vi "Boiler Controller.vi"() -> ()   [LabVIEW 2015]
uses:
  support/Message Queue/All Message Queues.ctl
  support/Message Queue/Message Cluster.ctl
  support/Message Queue/Message Queue.lvlib
panel:
  out "Error Out":errorcluster
  in  "Error In":errorcluster
  in  "Message Queues":T1
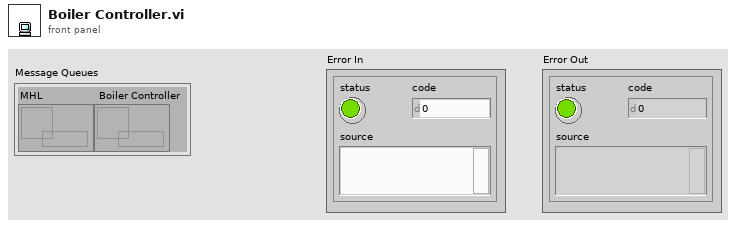
[diagram p1: front panel]
types:
  T1 = typedef "Message Queue.lvlib/All Message Queues.ctl" = cluster{"MHL":refnum<queue>, " Boiler Controller":refnum<queue>}
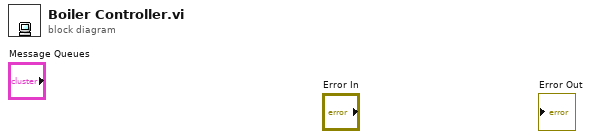
[diagram p0: block diagram]
diagram:
